vi "Dashboard Main.vi"() -> ()   [LabVIEW 2016]
uses:
  <vilib>/Utility/miscctls.llb/LVRowAndColumnTypeDef.ctl
  <vilib>/event_ctls.llb/eventvkey.ctl
  <vilib>/Rock Robotics/Network Tables/NT Read Boolean.vi
  <vilib>/Rock Robotics/WPI/Dashboard/WPI_DashboardLogging Global.vi
panel:
  out "timeLeft":dbl(slide) scale=0.0..150.0
  in  "TCP":refnum<k5>
  in  "Rec Mode":enum32{"Stop", "Record", "Playback"}(radio)
  out "Robot IP":string
  out "Image Message":string="Timeout in Camera Communications"
  in  "Dashboard Tab":T1(tab)
  out "Angle":dbl(knob) scale=-30.0..30.0
  out "Distance":dbl(slide)
  out "Shooter Speed":dbl(knob) scale=0.0..5600.0
  out "Climber State":u32(colorbox)
  out "Pressure":dbl(knob) scale=0.0..120.0
  out "NT Connection":bool
  out "Mode":T2(ring)=enum."Auto Disabled"
  out "Camera Info":cluster{"Mbps LED":bool, "Mbps":dbl, "fps":dbl} {"fps" format="%#.1g"; "Mbps" format="%#.1g"}
  in  "Autonomous Mode":i32(listbox)
  in  "Peg Side":i32(listbox)
  in  "RPM setting":dbl=5400.0
  out "gearLiftUp":bool
  out "gearLiftDown":bool
  out "gearClawOpen":bool
  out "Camera Image Right":T3(plugin-control)
  in  "DB/String 9":string
  in  "DB/String 8":string
  in  "DB/String 7":string
  in  "DB/String 6":string
  in  "DB/String 5":string
  in  "DB/String 4":string
  in  "DB/String 3":string
  in  "DB/String 2":string
  in  "DB/String 1":string
  in  "DB/String 0":string
  in  "DB/Slider 0":dbl(slide) scale=0.0..5.0
  in  "DB/Slider 1":dbl(slide) scale=0.0..5.0
  in  "DB/Slider 2":dbl(slide) scale=0.0..5.0
  in  "DB/Slider 3":dbl(slide) scale=0.0..5.0
  out "DB/LED 3":bool
  out "DB/LED 2":bool
  out "DB/LED 1":bool
  out "DB/LED 0":bool
  in  "DB/Button 3":bool
  in  "DB/Button 2":bool
  in  "DB/Button 1":bool
  in  "DB/Button 0":bool caption="New Name"
  in  "Camera Name":string(combo)="No Camera Selection"
  in  "Camera Settings":T4={"Frame Rate"=30, "Compression"=30, "Size"=1, "DB Camera Config"=FALSE} {"Frame Rate" scale=1.0..30.0; "Compression" scale=100.0..-1.0; "Size" items=["640x480", "320x240", "160x120"]}
  in  "Camera Name Right":string(combo)="No Camera Selection"
  in  "Camera Settings Right":T4={"Frame Rate"=30, "Compression"=30, "Size"=1, "DB Camera Config"=FALSE} {"Frame Rate" scale=1.0..30.0; "Compression" scale=100.0..-1.0; "Size" items=["640x480", "320x240", "160x120"]}
  in  "Test Slider":dbl(slide) scale=0.0..100.0 scale format="%#_3g"
  in  "On/Off":bool caption="Solenoid"
  in  "Test Name":u16(ring) items=["Select the test to run..."]
  in  "Test Tree":string(tree)
  in  "Motor":cluster{"Value":dbl, "Enable":bool} {"Value" scale=-1.0..1.0 scale format="%#_3g"}
  out "Progress":T5 {"Test Progress" scale=0.0..100.0}
  in  "Rev/Fwd":cluster{"Forward":bool, "Reverse":bool}
  in  "Test Ring":u16(ring) items=["Monochrome", "Color"]
  out "Cmd Status":string
  in  "Execute Command":bool
  in  "Command Params":string[][](table)
  in  "Command Selection":i32(listbox)
  in  "CheckList":i32(listbox)
  out "Tree":string(tree)
  out "Camera Image":T3(plugin-control)
  out "Background":bool
  # "Gear Claw"
  # "HW"
  # "HW"
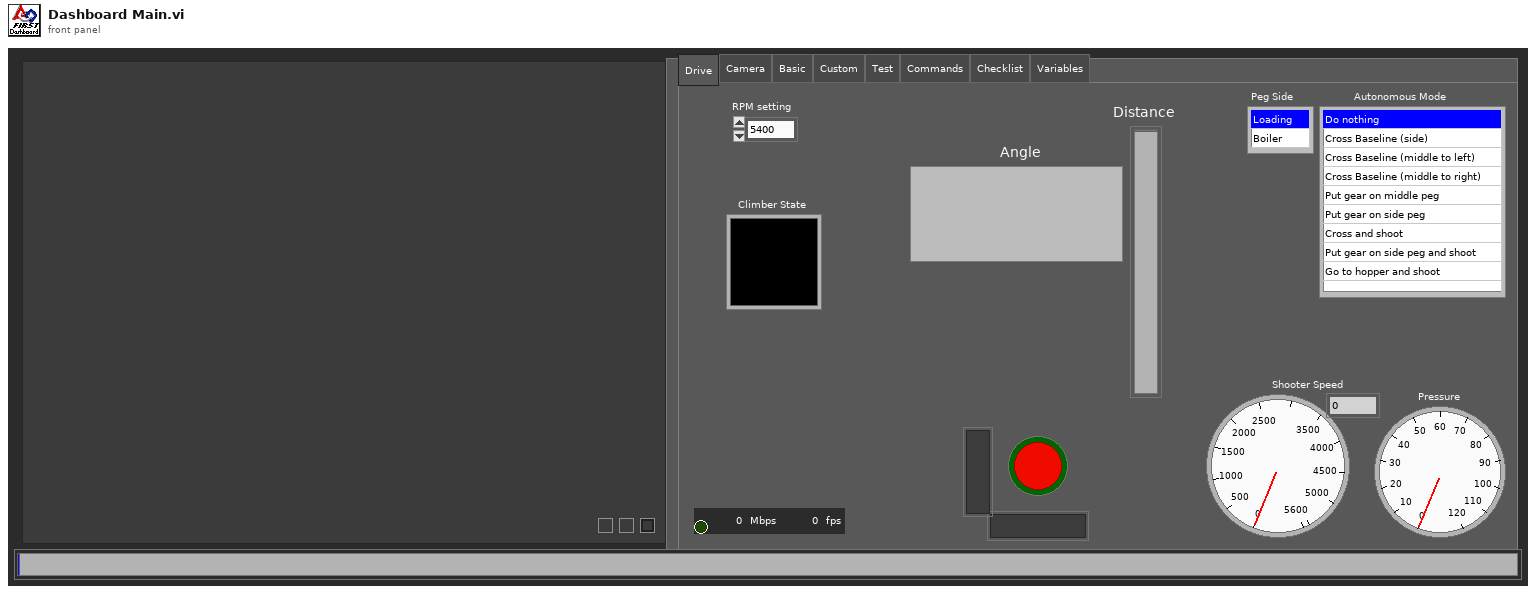
[diagram p1: front panel]
types:
  T1 = enum32{"Drive", "Camera", "Basic", "Custom", "Test", "Commands", "Checklist", "Variables"}
  T2 = enum8{"Tele-Op Disabled", "Tele-Op Enabled", "Auto Disabled", "Auto Enabled", "Test Disabled", "Test Enabled", "Disconnected", "No Code", "E-Stop"}
  T3 = typedef "IMAQ Image.ctl" = refnum<image>
  T4 = cluster{"Frame Rate":i32, "Compression":i32, "Size":u16, "DB Camera Config":bool}
  T5 = cluster{"Test Progress":u8, "Test Progress Text":string}
  T6 = typedef "Image Type" = u32
  T7 = cluster{"IDs":cluster{"RPC field ID":u16, "Unique ID":u16}, "String":string}
  T8 = enum32{"Drive", "Basic", "Custom", "Test", "Checklist", "Variables"}
  T9 = cluster{"Error Strings":string, "Disable Counts":cluster{u16, u16}, "Rail Faults":cluster{u16, u16, u16}, "Robot IP":string, "DB Mode":u8, "Event Info":cluster{"Name":string, "Type":u8, "Number":u16, "Replay":u8}}
  T10 = cluster{"Storage":cluster{"Disk Free":u64, "RAM Block":u32, "RAM free":u32}, "CPU Utilization":cluster{"CPU % ISR":sgl, "CPU % Time Crit":sgl, "CPU % Timed Str":sgl, "CPU % High":sgl, "CPU % Above":sgl, "CPU % Normal":sgl, "CPU % Low":sgl}, "CAN":cluster{"% Bus Utilization":sgl, "Bus Off Cnt":u32, "TX_FIFO Full Cnt":u32, "Receive Error Cnt":u8, "Transmit Error Cnt":u8}, "HID":cluster{"HID Outputs":u32, "Rumble Low":u16, "Rumble High":u16}[]}
  T11 = cluster{"Status bits":cluster{"Test Mode":bool, "Autonomous":bool, "Enabled":bool, "Code Start":bool, "Brownout":bool, "Reserved 2":bool, "Reserved 3":bool, "E-Stop":bool}, "Code Trace":cluster{"Disabled":bool, "TeleOp":bool, "Auto":bool, "Test":bool}, "Controller Type":enum16{"unknown", "cRIO", "roboRio"}, "Code?":enum16{"unknown", "noCode", "code"}, "Battery V":dbl}
  T12 = cluster{"Control Bits":cluster{"TestMode":bool, "Autonomous":bool, "Enabled":bool, "FMS Present":bool, bool, bool, bool, "E-Stop":bool}, "Team Station ":u8, "Countdown":sgl, "Joystick Values":cluster{"Axes":dbl[], "Buttons":bool[], "POVs":i16[]}[]}
  T13 = cluster{"Camera Image":refnum<vi>, "Dashboard Tab":refnum<vi>, "Background":refnum<vi>, "Rec Mode":refnum<vi>, "Test Slider":refnum<vi>, "On/Off ":refnum<vi>, "Test Ring":refnum<vi>, "Rev/Fwd":refnum<vi>, "Test Name":refnum<vi>, "Motor":refnum<vi>, "Progress":refnum<vi>, "CheckList":refnum<vi>, "Tree":refnum<vi>, "Test Tree":refnum<vi>, "Command Params":refnum<vi>, "Command Selection":refnum<vi>, "Execute Command":refnum<vi>, "Cmd Status":refnum<vi>, "Camera Settings":refnum<vi>, "Camera Name":refnum<vi>, "Camera Info":refnum<vi>, "Camera Settings Right":refnum<vi>, "Camera Name Right":refnum<vi>, "Camera Image Right":refnum<vi>}
  T14 = cluster{"Operation":enum16{"Update", "Clear"}, "Color Box":u32}[]
  T15 = typedef "eventvkey.ctl" = enum16{"ASCII", "Enter", "Return", "Shift", "Ctrl", "Alt", "Cmd", "Opt", "Caps", "NumLock", "Clear", "Break", "Up", "Down", "Left", "Right", "Insert", "Delete", "Home", "End", "PageUp", "PageDown", "Escape", "Help", "Pause", "ScrollLock", "F1", "F2", "F3", "F4", "F5", "F6", "F7", "F8", "F9", "F10", "F11", "F12", "F13", "F14", "F15", "F16", "F17", "F18", "F19", "F20", "F21", "F22", "F23", "F24", "Play", "VolumeUp", "VolumeDown", "Mute", "Two Byte Char"}
  T16 = cluster{"Image Size":bool, "Image Type":bool, "Pixel Value":bool, "ROI Information":bool, "Zoom Factor":bool}
  T17 = cluster{"Operation":enum16{"Update", "Clear"}, "Color Box":u32}
  T18 = typedef "LVRowAndColumnTypeDef.ctl" = cluster{"Row":i32, "Column":i32}
  T19 = cluster{"Shift":bool, "Ctrl":bool, "Alt":bool, "Cmd":bool, "Opt":bool}
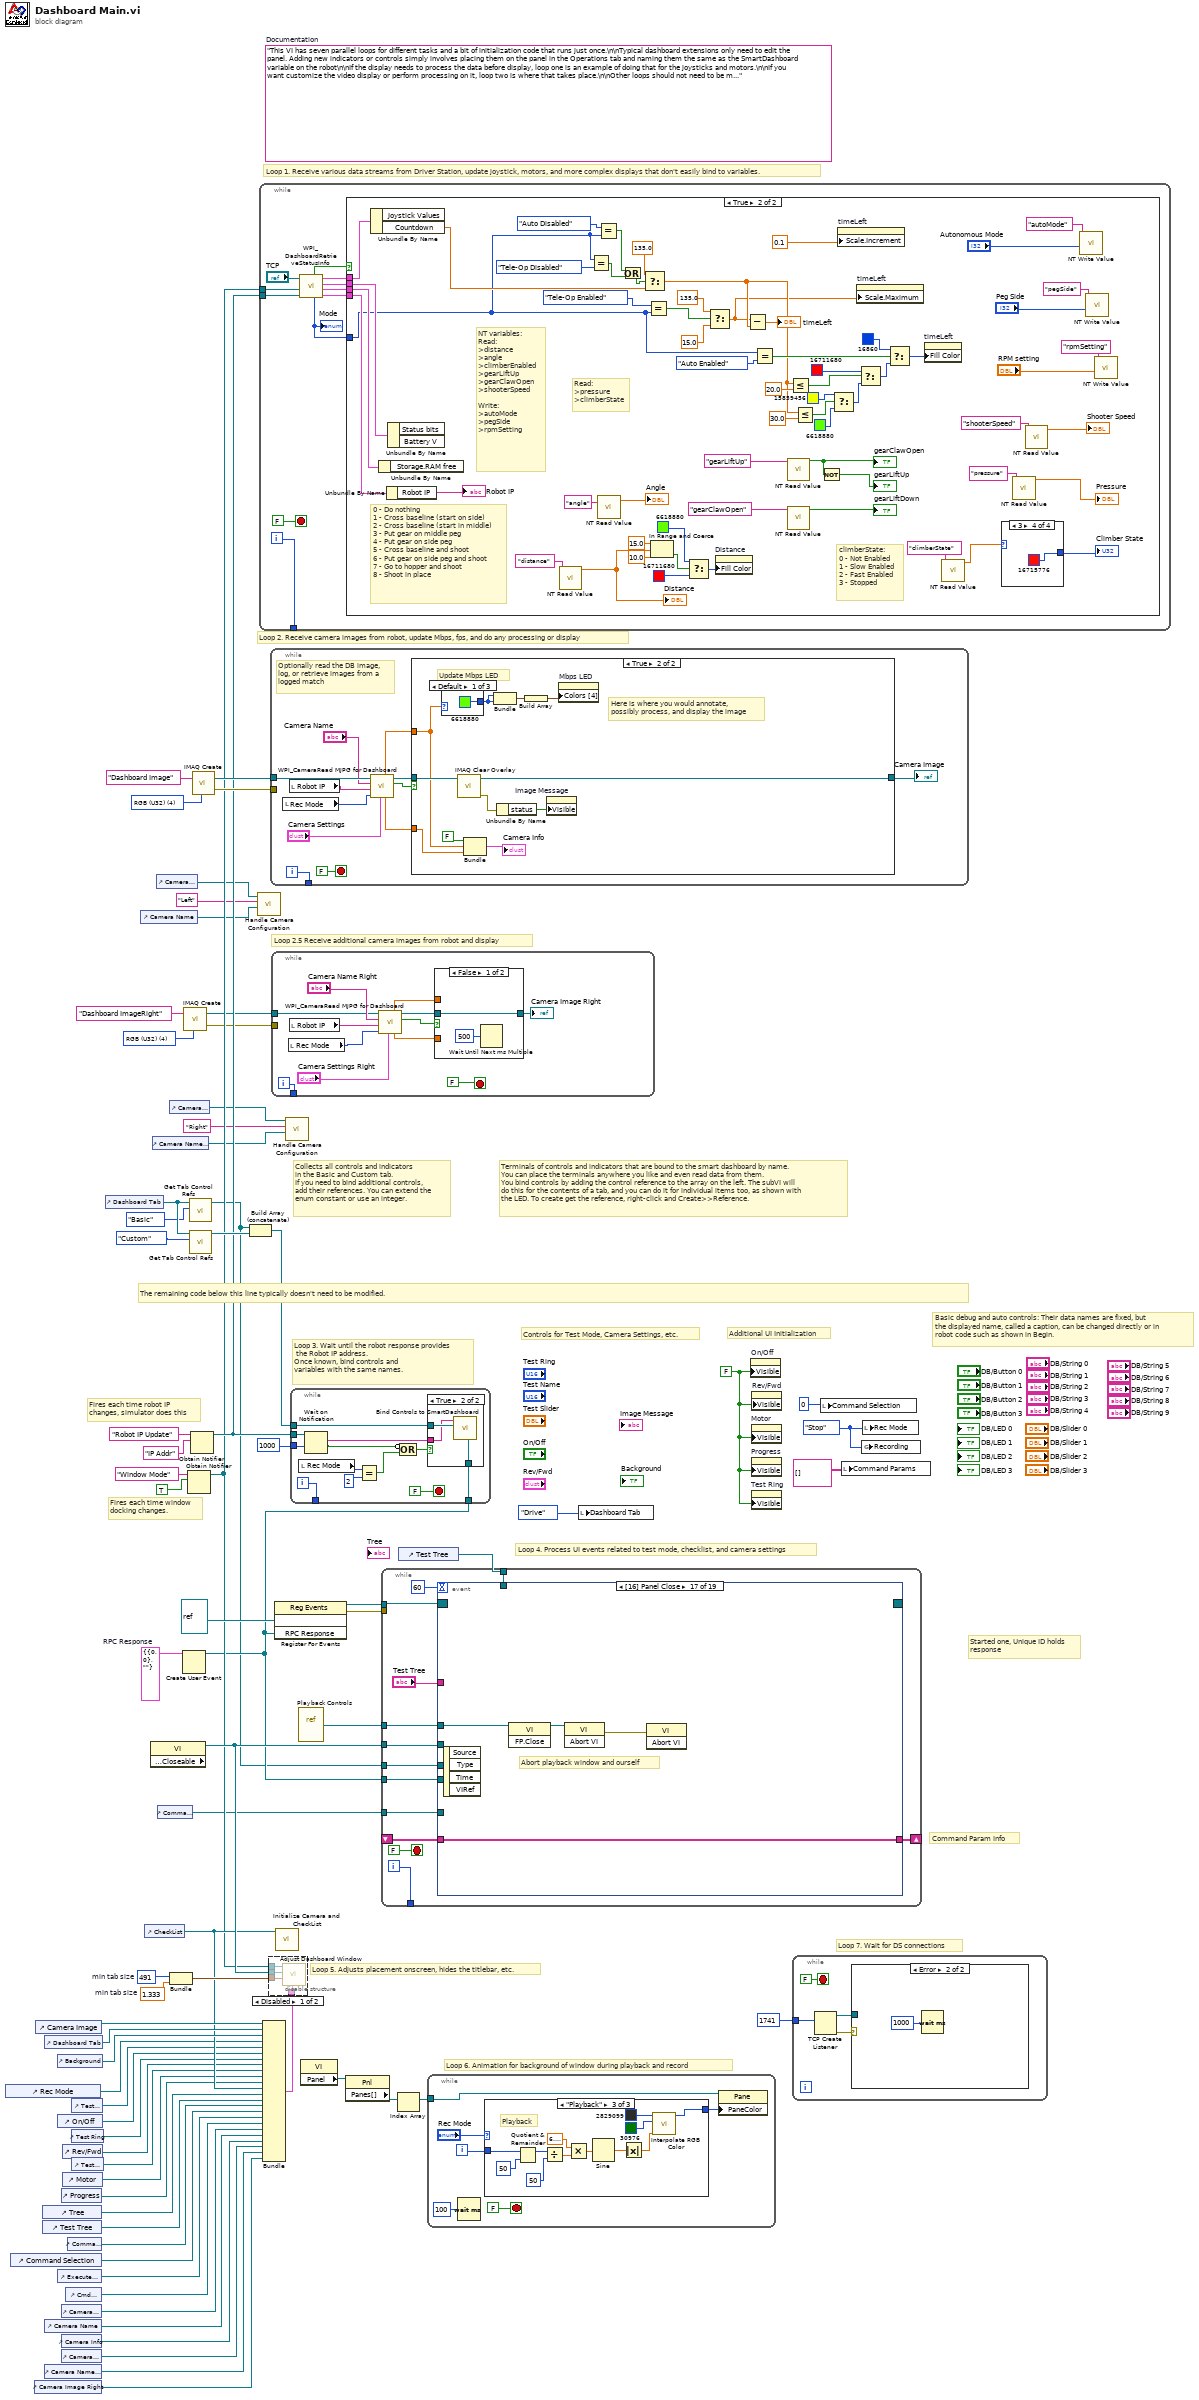
[diagram p0: block diagram]
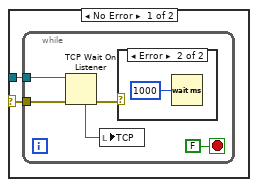
[diagram p4: hidden frame]
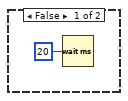
[diagram p6: hidden frame]
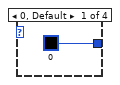
[diagram p7: hidden frame]
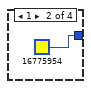
[diagram p8: hidden frame]
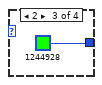
[diagram p9: hidden frame]
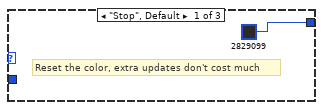
[diagram p10: hidden frame]
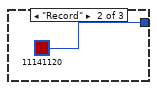
[diagram p11: hidden frame]
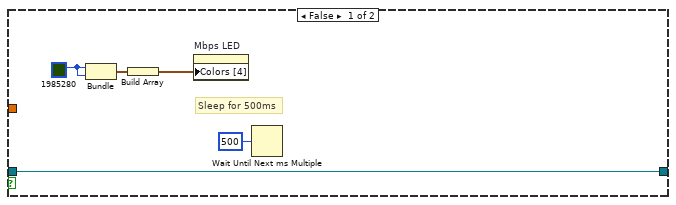
[diagram p13: hidden frame]
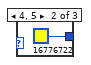
[diagram p14: hidden frame]
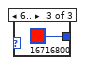
[diagram p15: hidden frame]
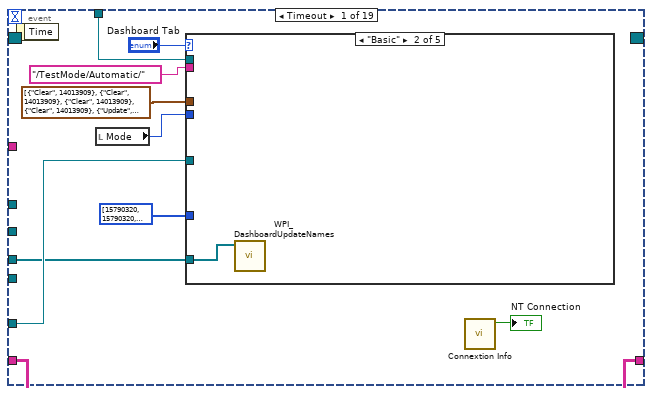
[diagram p16: hidden frame]
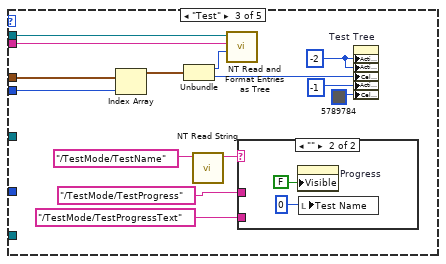
[diagram p18: hidden frame]
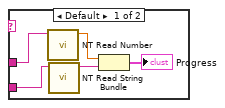
[diagram p19: hidden frame]
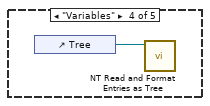
[diagram p20: hidden frame]
diagram:
  w10 = T6 4 items=["Grayscale (U8)", "Grayscale (I16)", "Grayscale (SGL)", "Complex (CSG)", "RGB (U32)", "HSL (U32)", "RGB (U64)"] ("Image Type")
  w24 = T7 {"IDs"={"RPC field ID"=0, "Unique ID"=0}, "String"=""}  # RPC Response
  w49 = 491  # min tab size
  w48 = 1.333  # min tab size
  w56 = enum32{"Stop", "Record", "Playback"}."Stop" ("Rec Mode")
  w31 = FALSE ("Visible")
  (unwired) "This VI has seven parallel loops for different tasks and a bit of initialization code that runs just once.\n\nTypical dashboard extensions only need to edit the panel. Adding new indicators or controls simply involves placing them on the panel in the Operations tab and naming them the same as the SmartDashboard variable on the robot\n\nIf the display needs to process the data before display, loop one is an example of doing that for the joysticks and motors.\n\nIf you want customize the video display or perform processing on it, loop two is where that takes place.\n\nOther loops should not need to be modified. They are pretty standard, and document the task they perform."  # Documentation
  w73 = T6 4 items=["Grayscale (U8)", "Grayscale (I16)", "Grayscale (SGL)", "Complex (CSG)", "RGB (U32)", "HSL (U32)", "RGB (U64)"] ("Image Type")
  # "Loop 2.5 Receive additional camera images from robot and display"
  # "Command Param Info"
  # "Started one, Unique ID holds\nresponse"
  # "Loop 7. Wait for DS connections"
  # "Basic debug and auto controls: Their data names are fixed, but\nthe displayed name, called a caption, can be changed directly or in\nrobot code such as shown in Begin."
  # "Controls for Test Mode, Camera Settings, etc."
  # "Additional UI Initialization"
  # "Loop 6. Animation for background of window during playback and record"
  # "Fires each time robot IP\nchanges, simulator does this"
  # "Fires each time window\ndocking changes."
  # "Collects all controls and indicators\nin the Basic and Custom tab.\nIf you need to bind additional controls,\nadd their references. You can extend the\nenum constant or use an integer."
  # "The remaining code below this line typically doesn't need to be modified."
  # "Loop 4. Process UI events related to test mode, checklist, and camera settings"
  # "Terminals of controls and indicators that are bound to the smart dashboard by name.\nYou can place the terminals anywhere you like and even read data from them.\nYou bind controls by adding the control reference to the array on the left. The subVI will\ndo this for the contents of a tab, and you can do it for individual items too, as shown with\nthe LED. To create get the reference, right-click and Create>>Reference."
  # "Loop 3. Wait until the robot response provides\n the Robot IP address.\nOnce known, bind controls and\nvariables with the same names."
  # "Loop 5. Adjusts placement onscreen, hides the titlebar, etc."
  # "Loop 1. Receive various data streams from Driver Station, update joystick, motors, and more complex displays that don't easily bind to variables."
  # "Loop 2. Receive camera images from robot, update Mbps, fps, and do any processing or display"
  n1 = control-ref of="Rec Mode"() -> (w37:refnum<vi>)
  n2 = control-ref of="Command Selection"() -> (w23:refnum<vi>)
  n3 = control-ref of="Camera Image Right"() -> (w1:refnum<vi>)
  n4 = control-ref of="Camera Image"() -> (w51:refnum<vi>)
  n5 = control-ref of="Tree"() -> (w41:refnum<vi>)
  n6 = control-ref of="Test Tree"() -> (w40:refnum<vi>)
  n7 = control-ref of="Dashboard Tab"() -> (w50:refnum<vi>)
  n8 = control-ref of="Camera Name"() -> (w14:refnum<vi>)
  n9 = control-ref of="Camera Name Right"() -> (w2:refnum<vi>)
  n10 = control-ref of="Execute Command"() -> (w25:refnum<vi>)
  n11 = control-ref of="Background"() -> (w46:refnum<vi>)
  n12 = control-ref of="On/Off"() -> (w35:refnum<vi>)
  n13 = control-ref of="Progress"() -> (w32:refnum<vi>)
  n14 = control-ref of="Camera Settings"() -> (w15:refnum<vi>)
  n15 = control-ref of="Camera Info"() -> (w13:refnum<vi>)
  n16 = control-ref of="Camera Settings Right"() -> (w3:refnum<vi>)
  n17 = control-ref of="Rev/Fwd"() -> (w33:refnum<vi>)
  n18 = control-ref of="Motor"() -> (w38:refnum<vi>)
  n19 = control-ref of="Cmd Status"() -> (w19:refnum<vi>)
  n20 = control-ref of="Command Params"() -> (w26:refnum<vi>)
  n21 = control-ref of="Test Slider"() -> (w36:refnum<vi>)
  n22 = control-ref of="Test Ring"() -> (w34:refnum<vi>)
  n23 = control-ref of="Test Name"() -> (w39:refnum<vi>)
  n24 = control-ref of="Dashboard Tab"() -> (w54:refnum<vi>)
  n25 = control-ref of="Camera Name"() -> (w16:refnum<vi>)
  n26 = control-ref of="CheckList"() -> (w42:refnum<vi>)
  n27 = property class="VI" props=["Front Panel.Closeable"]() -> (reference out=w55:refnum<vi>)  [unwired: 2 in, 2 out]
  n28 = control-ref of="Camera Name Right"() -> (w6:refnum<vi>)
  n29 = control-ref of="Camera Settings"() -> (w17:refnum<vi>)
  n30 = control-ref of="Command Params"() -> (w18:refnum<vi>)
  n31 = control-ref of="Camera Settings Right"() -> (w7:refnum<vi>)
  n32 = Bundle("min tab size"=w49, "min tab size"=w48) -> (w47:cluster{"min tab size":i32, "min tab size":dbl})  [unwired: 1 in]
  n33 = Create User Event(user event datatype=w24) -> (user event=w20:refnum<user-event>)  [unwired: 1 in, 1 out]
  n34 = call "IMAQ Create"("Image Name"="Dashboard ImageRight", "Image Type"=w10) -> ("New Image"=w9:T3, "error out"=w8:errorcluster)  [unwired: 2 in, 1 out]
  n35 = Obtain Notifier(name (unnamed)="Window Mode", notification data type=TRUE) -> (notifier out=w29:refnum<notifier>)  [unwired: 2 in, 2 out]
  n36 = call <vilib>:"Get Tab Control Refs.vi"("Page Index"=T8."Basic" ("Dashboard Tab"), "TabControl in"=w54) -> ("ControlsOnPage"=w12:refnum<vi>[])  [unwired: 9 in]
  n37 = call <vilib>:"Get Tab Control Refs.vi"("Page Index"=T8."Custom" ("Dashboard Tab"), "TabControl in"=w54) -> ("ControlsOnPage"=w53:refnum<vi>[])  [unwired: 9 in]
  n38 = Obtain Notifier(name (unnamed)="Robot IP Update", notification data type="IP Addr" ("name (unnamed)")) -> (notifier out=w30:refnum<notifier>)  [unwired: 2 in, 2 out]
  n39 = call "IMAQ Create"("Image Name"="Dashboard Image", "Image Type"=w73) -> ("New Image"=w71:T3, "error out"=w70:errorcluster)  [unwired: 2 in, 1 out]
  n40 = Build Array (concatenate)(w12, w53) -> (w52:refnum<vi>[])
  n41 = call "Handle Camera Configuration.vi"("CameraNameRef"=w16, "Camera File Name"="Left", "ClusterRef"=w17) -> ()  [unwired: 9 in]
  n42 = while {
    tunnel: [w83] -> _
    tunnel: w30 -> [w77]
    tunnel: w29 -> [w74]
    i -> [w83]
    stop <- FALSE stop-if-true
    n43 = call <vilib>:"WPI_DashboardRetrieveStatusInfo.vi"("Binding Refnum"=w77, "Window Mode Notifier"=w74, "TCP Cnx"="TCP") -> ("Power and Errors"=w78:T9, "Robot Metrics"=w81:T10, "Status Info"=w82:T11, "Control Info"=w79:T12, "Robot Mode"=w76:T2, "Process?"=w80:bool)  [unwired: 3 in]
    "Mode" <- w76
    n44 = case shown="True" w80 {
      tunnel: w82 -> [_ w147]
      tunnel: w81 -> [_ w146]
      tunnel: w79 -> [_ w145]
      tunnel: w78 -> [_ w144]
      tunnel: w76 -> [_ w114]
      frame False {
        n45 = Wait (ms)(milliseconds to wait=u32 20) -> ()  [unwired: 1 out]
      }
      frame True {
        # "climberState:\n0 - Not Enabled\n1 - Slow Enabled\n2 - Fast Enabled\n3 - Stopped"
        # "Read:\n>pressure\n>climberState"
        # "0 - Do nothing\n1 - Cross baseline (start on side)\n2 - Cross baseline (start in middle)\n3 - Put gear on middle peg\n4 - Put gear on side peg\n5 - Cross baseline and shoot\n6 - Put gear on side peg and shoot\n7 - Go to hopper and shoot\n8 - Shoot in place"
        # "NT variables:\nRead:\n>distance\n>angle\n>climberEnabled\n>gearLiftUp\n>gearClawOpen\n>shooterSpeed\n\nWrite:\n>autoMode\n>pegSide\n>rpmSetting"
        n46 = Unbundle By Name(w145) -> ("Countdown"=w115:sgl)  [unwired: 1 out]
        n47 = Unbundle By Name(w146) -> ()  [unwired: 1 out]
        n48 = Unbundle By Name(w144) -> ("Robot IP"=→"Robot IP":string)
        n49 = Unbundle By Name(w147) -> ()  [unwired: 2 out]
        n50 = call-poly <vilib>:"NT Read Value.vi"("Name"="distance") -> ("Numeric"=w90:dbl)  [unwired: 9 in, 1 out]
        "Distance" <- w90
        n51 = Equal?(x=w114, y=T2."Tele-Op Disabled") -> (x = y?=w118:bool)
        n52 = Equal?(x=T2."Auto Disabled" ("Robot Mode"), y=w114) -> (x = y?=w119:bool)
        n53 = call-poly <vilib>:"NT Read Value.vi"("Name"="angle") -> ("Numeric"=→"Angle":dbl)  [unwired: 9 in, 1 out]
        n54 = Or(x=w119, y=w118) -> (x .or. y?=w120:bool)
        n55 = Select(t=sgl 135.0, s=w120, f=w115) -> (s? t:f=w124:sgl)
        n56 = Equal?(x=T2."Tele-Op Enabled" ("Robot Mode"), y=w114) -> (x = y?=w126:bool)
        n57 = In Range and Coerce(upper limit=15.0, x=w90, lower limit=10.0) -> (In Range?=w93:bool)  [unwired: 1 out]
        n58 = Select(t=u32 6618880, s=w93, f=u32 16711680) -> (s? t:f=w94:u32)
        n59 = Select(t=135.0, s=w126, f=15.0) -> (s? t:f=w122:dbl)
        n60 = property on="Distance" class="Slide (strict)"("Fill Color"=w94) -> ()  [unwired: 2 in, 2 out]
        n61 = Subtract(x=w122, y=w124) -> (x-y=→"timeLeft":dbl)
        n62 = Equal?(x=w114, y=T2."Auto Enabled") -> (x = y?=w137:bool)
        n63 = call-poly <vilib>:"NT Read Value.vi"("Name"="gearLiftUp") -> ("Boolean"=w98:bool)  [unwired: 9 in, 1 out]
        "gearClawOpen" <- w98
        n64 = call-poly <vilib>:"NT Read Value.vi"("Name"="gearClawOpen") -> ("Boolean"=→"gearLiftDown":bool)  [unwired: 9 in, 1 out]
        n65 = Less Or Equal?(x=w124, y=sgl 20.0) -> (x <= y?=w116:bool)
        n66 = Less Or Equal?(x=w124, y=sgl 30.0) -> (x <= y?=w129:bool)
        n67 = Not(x=w98) -> (.not. x?=→"gearLiftUp":bool)
        n68 = Select(t=u32 15859456, s=w129, f=u32 6618880) -> (s? t:f=w130:u32)
        n69 = property on="timeLeft" class="Slide (strict)"("Scale.Increment"=0.1 ("Scale.Range:Increment")) -> ()  [unwired: 2 in, 2 out]
        n70 = property on="timeLeft" class="Slide (strict)"("Scale.Maximum"=w122) -> ()  [unwired: 2 in, 2 out]
        n71 = Select(t=u32 16711680, s=w116, f=w130) -> (s? t:f=w132:u32)
        n72 = Select(t=u32 16860, s=w137, f=w132) -> (s? t:f=w135:u32)
        n73 = property on="timeLeft" class="Slide (strict)"("Fill Color"=w135) -> ()  [unwired: 2 in, 2 out]
        n74 = call-poly <vilib>:"NT Read Value.vi"("Name"="climberState") -> ("Numeric"=w106:dbl)  [unwired: 9 in, 1 out]
        n75 = case shown="3" w106 {
          tunnel: [u32 0 ("Climber State") u32 16775954 ("Climber State") u32 1244928 ("Climber State") u32 16715776 ("Climber State")] -> w105
          frame 0, Default {
          }
          frame 1 {
          }
          frame 2 {
          }
          frame 3 {
          }
        }
        "Climber State" <- w105
        n76 = call-poly <vilib>:"NT Read Value.vi"("Name"="pressure") -> ("Numeric"=→"Pressure":dbl)  [unwired: 9 in, 1 out]
        n77 = call-poly <vilib>:"NT Read Value.vi"("Name"="shooterSpeed") -> ("Numeric"=→"Shooter Speed":dbl)  [unwired: 9 in, 1 out]
        n78 = call-poly <vilib>:"NT Write Value.vi"("Numeric"="Autonomous Mode", "Name"="autoMode") -> ()  [unwired: 9 in, 1 out]
        n79 = call-poly <vilib>:"NT Write Value.vi"("Numeric"="Peg Side", "Name"="pegSide") -> ()  [unwired: 9 in, 1 out]
        n80 = call-poly <vilib>:"NT Write Value.vi"("Numeric"="RPM setting", "Name"="rpmSetting") -> ()  [unwired: 9 in, 1 out]
      }
    }
  }
  n81 = Bundle("Camera Image"=w51, "Dashboard Tab"=w50, "Background"=w46, "Rec Mode"=w37, "Test Slider"=w36, "On/Off"=w35, "Test Ring"=w34, "Rev/Fwd"=w33, "Test Name"=w39, "Motor"=w38, "Progress"=w32, "CheckList"=w42, "Tree"=w41, "Test Tree"=w40, "Command Params"=w26, "Command Selection"=w23, "Execute Command"=w25, "Cmd Status"=w19, "Camera Settings"=w15, "Camera Name"=w14, "Camera Info"=w13, "Camera Settings Right"=w3, "Camera Name Right"=w2, "Camera Image Right"=w1) -> (w43:T13)  [unwired: 1 in]
  n82 = disable-structure shown="Disabled" {
    disable-tunnel: w55 -> [w155 _]
    disable-tunnel: w47 -> [w154 _]
    disable-tunnel: w43 -> [w153 _]
    disable-tunnel: w29 -> [w152 _]
    frame Disabled {
      n83 = call "Adjust Dashboard Window.vi"("Sizing Refnums"=w153, "Size Constraints"=w154, "VI"=w155, "WIn Mode"=w152) -> ()  [unwired: 8 in]
    }
    frame Enabled {
    }
  }
  n84 = while {
    tunnel: w71 -> [w165]
    tunnel: w70 -> [_]
    tunnel: [w166] -> _
    i -> [w166]
    stop <- FALSE stop-if-true
    # "Optionally read the DB image,\nlog, or retrieve images from a\nlogged match"
    n85 = local read "Rec Mode"() -> (w161:enum32{"Stop", "Record", "Playback"})
    n86 = local read "Robot IP"() -> (w160:string)
    n87 = call <vilib>:"WPI_CameraRead MJPG for Dashboard.vi"("Camera Settings"="Camera Settings", "Rec Mode"=w161, "Robot IP"=w160, "Camera Name"="Camera Name", "Refnum in"=w165) -> ("Active"=w163:bool, "Refnum out"=w164:T3, "FPS"=w162:dbl, "Bandwidth (Mbps)"=w159:dbl)  [unwired: 3 in]
    n88 = case shown="True" w163 {
      tunnel: w164 -> [w168 w179]
      tunnel: w159 -> [_ w176]
      tunnel: w162 -> [_ w177]
      tunnel: [w168 w173] -> w156
      frame False {
        w170 = u32 1985280 ("Color Box")
        # "Sleep for 500ms"
        n89 = Bundle("Color Box"=w170, "Color Box"=w170) -> (w171:cluster{"Color Box":u32, "Color Box":u32})  [unwired: 1 out]
        n90 = Build Array(w171) -> (w169:cluster{"Color Box":u32, "Color Box":u32}[])
        n91 = property on="Mbps LED" class="Bool (strict)"("Colors [4]"=w169) -> ()  [unwired: 2 in, 2 out]
        n92 = Wait Until Next ms Multiple(millisecond multiple=u32 500) -> ()  [unwired: 1 out]
      }
      frame True {
        # "Here is where you would annotate,\npossibly process, and display the image"
        # "Update Mbps LED"
        n93 = case shown="Default" w176 {
          tunnel: [u32 6618880 ("Color Box") u32 16776722 ("Color Box") u32 16716800 ("Color Box")] -> w180
          frame Default {
          }
          frame 4, 5 {
          }
          frame 6.. {
          }
        }
        n94 = call "IMAQ Clear Overlay"("Image"=w179) -> ("error out"=w182:errorcluster, "Image Out"=w173:T3)  [unwired: 2 in, 7 out]
        n95 = Bundle(FALSE, "Bandwidth (Mbps)"=w176, "FPS"=w177) -> (→"Camera Info":cluster{bool, "Bandwidth (Mbps)":dbl, "FPS":dbl})  [unwired: 1 in]
        n96 = Bundle("Color Box"=w180, "Color Box"=w180) -> (w181:cluster{"Color Box":u32, "Color Box":u32})  [unwired: 1 out]
        n97 = Unbundle By Name(w182) -> ("status"=w183:bool)
        n98 = Build Array(w181) -> (w178:cluster{"Color Box":u32, "Color Box":u32}[])
        n99 = property on="Image Message" class="Str"("Visible"=w183) -> ()  [unwired: 2 in, 2 out]
        n100 = property on="Mbps LED" class="Bool (strict)"("Colors [4]"=w178) -> ()  [unwired: 2 in, 2 out]
      }
    }
    "Camera Image" <- w156
  }
  n101 = while {
    tunnel: w9 -> [w197]
    tunnel: w8 -> [_]
    tunnel: [w191] -> _
    i -> [w191]
    stop <- FALSE stop-if-true
    n102 = local read "Rec Mode"() -> (w195:enum32{"Stop", "Record", "Playback"})
    n103 = local read "Robot IP"() -> (w196:string)
    n104 = call <vilib>:"WPI_CameraRead MJPG for Dashboard.vi"("Camera Settings"="Camera Settings Right", "Rec Mode"=w195, "Robot IP"=w196, "Camera Name"="Camera Name Right", "Refnum in"=w197) -> ("Active"=w190:bool, "Refnum out"=w193:T3, "FPS"=w188:dbl, "Bandwidth (Mbps)"=w189:dbl)  [unwired: 3 in]
    n105 = case shown="False" w190 {
      tunnel: w193 -> [w199 w201]
      tunnel: w189 -> [_ _]
      tunnel: w188 -> [_ _]
      tunnel: [w199 w201] -> w187
      frame False {
        n106 = Wait Until Next ms Multiple(millisecond multiple=u32 500) -> ()  [unwired: 1 out]
      }
      frame True {
      }
    }
    "Camera Image Right" <- w187
  }
  n107 = register-events(refnum<vi> refnum, w20) -> (reference out=w60:refnum<event-registration>, error out=w59:errorcluster)  [unwired: 2 in]
  n108 = call "Initialize Camera and CheckList.vi"("ListBox in"=w42) -> ()  [unwired: 11 in]
  n109 = call "Handle Camera Configuration.vi"("CameraNameRef"=w6, "Camera File Name"="Right", "ClusterRef"=w7) -> ()  [unwired: 9 in]
  n110 = while {
    tunnel: w52 -> [w213]
    tunnel: w30 -> [w211]
    tunnel: [w209] -> _
    tunnel: u32 1000 ("milliseconds to wait") -> [w208]
    tunnel: w20 -> [w202]
    i -> [w209]
    stop <- FALSE stop-if-true
    n111 = local read "Rec Mode"() -> (w204:enum32{"Stop", "Record", "Playback"})
    n112 = Wait on Notification(notifier=w211, timeout in ms (-1)=w208) -> (notification=w210:string, timed out?=w206:bool)  [unwired: 2 in, 2 out]
    n113 = Equal?(x=w204, y=u16 2 ("Rec Mode")) -> (x = y?=w205:bool)
    n114 = Compound Arithmetic op=OR(invert w206, w205) -> (w207:bool)
    n115 = case shown="True" w207 {
      tunnel: w213 -> [_ w216]
      tunnel: w210 -> [_ w215]
      tunnel: w202 -> [_ w214]
      frame False {
      }
      frame True {
        n116 = call <vilib>:"Bind Controls to SmartDashboard.vi"("RPC ref"=w214, "Bound Control Refs"=w216, "Server IP Address"=w215) -> ()  [unwired: 9 in]
      }
    }
  }
  n117 = vi-ref "Playback Controls.vi"() -> (w61:refnum<vi>)
  n118 = property class="VI"() -> ("Panel"=w63:refnum<vi>)  [unwired: 2 in, 2 out]
  n119 = property class="Pnl"(reference=w63) -> ("Panes[]"=w64:refnum<vi>[])  [unwired: 1 in, 2 out]
  n120 = Index Array(array=w64) -> (element=w62:refnum<vi>)  [unwired: 1 in]
  n121 = control-ref of="Test Tree"() -> (w65:refnum<vi>)
  n122 = while {
    tunnel: [w226] -> _
    tunnel: w65 -> [w225]
    tunnel: w61 -> [w224]
    tunnel: w60 -> [w223]
    tunnel: w59 -> [_]
    tunnel: w55 -> [w222]
    tunnel: w20 -> [w221]
    tunnel: w18 -> [w220]
    shift-right: [w219] -> _
    shift-left: _ -> [w218]
    tunnel: w12 -> [w217]
    i -> [w226]
    stop <- FALSE stop-if-true
    n123 = event shown="[16] Panel Close" {
      selector: w223 -> [_ _ _ _ _ _ _ _ _ _ _ _ _ _ _ _ _ _ _]
      dyn-events: [_ _ _ _ _ _ _ _ _ _ _ _ _ _ w476 _ _ _ _] -> _
      timeout: u32 60 ("milliseconds to wait") -> [_ _ _ _ _ _ _ _ _ _ _ _ _ _ _ _ _ _ _]
      tunnel: w225 -> [w238 _ _ _ _ _ _ _ _ _ _ _ _ _ _ _ _ _ _]
      tunnel: "Test Tree" -> [_ _ _ _ _ _ _ _ _ w443 w451 w453 w457 w465 _ _ _ _ _]
      tunnel: w224 -> [_ _ _ _ _ _ _ _ _ _ _ _ _ _ w478 _ w496 _ _]
      tunnel: w222 -> [_ _ _ _ _ _ _ _ _ _ _ _ _ _ w474 _ _ _ _]
      tunnel: w221 -> [_ _ _ _ _ _ _ _ _ _ _ _ _ _ w470 _ _ _ _]
      tunnel: w220 -> [w233 _ _ _ w394 _ _ _ _ _ _ _ _ _ _ _ _ _ _]
      tunnel: [w232 w277 w379 w384 w392 w401 w411 w418 w430 w442 w449 w452 w456 w464 w469 w491 w493 w497 w508] -> w219
      tunnel: w218 -> [w232 w277 w379 w384 w392 _ _ w418 w430 w442 w449 w452 w456 w464 w469 w491 w493 w497 w508]
      tunnel: w217 -> [w230 _ _ _ _ _ _ _ _ _ _ _ _ _ _ _ _ _ _]
      event Timeout {
        n124 = event-data() -> ()  [unwired: 1 in, 1 out]
        n125 = local read "Mode"() -> (w235:T2)
        n126 = case shown="\"Basic\"" "Dashboard Tab" {
          tunnel: w238 -> [_ _ w254 _ _]
          tunnel: "/TestMode/Automatic/" ("Name Pattern") -> [_ _ w253 _ _]
          tunnel: T14 [{"Operation"=enum."Clear", "Color Box"=14013909}, {"Operation"=enum."Clear", "Color Box"=14013909}, {"Operation"=enum."Clear", "Color Box"=14013909}, {"Operation"=enum."Clear", "Color Box"=14013909}, {"Operation"=enum."Update", "Color Box"=14013909}, {"Operation"=enum."Update", "Color Box"=16777215}, {"Operation"=enum."Clear", "Color Box"=14013909}, {"Operation"=enum."Clear", "Color Box"=14013909}, {"Operation"=enum."Clear", "Color Box"=14013909}] -> [_ _ w246 _ w270]
          tunnel: w235 -> [_ _ w245 _ w269]
          tunnel: u32[] [15790320, 15790320, 15790320, 15790320, 16777215, 16777215, 15790320, 15790320, 15790320] -> [_ _ _ _ w275]
          tunnel: w233 -> [_ _ _ _ w263]
          tunnel: w230 -> [_ w240 _ _ _]
          frame "Custom", Default {
          }
          frame "Basic" {
            n127 = call <vilib>:"WPI_DashboardUpdateNames.vi"("Controls on Tab"=w240) -> ()  [unwired: 11 in]
          }
          frame "Test" {
            w252 = -2 ("Active Item:Row Number")
            n128 = Index Array(array=w246, index=w245) -> (element=w247:T17)
            n129 = Unbundle(w247) -> ("Operation"=w248:enum16{"Update", "Clear"}, "Color Box"=w249:u32)
            n130 = call <vilib>:"NT Read String.vi"("Name"="/TestMode/TestName") -> ("String"=w243:string)  [unwired: 9 in, 1 out]
            n131 = call <vilib>:"NT Read and Format Entries as Tree.vi"("Operation"=w248, "Name Pattern"=w253, "Tree Refnum"=w254) -> ()  [unwired: 7 in, 2 out]
            n132 = case shown="\"\"" w243 {
              tunnel: "/TestMode/TestProgress" ("Name") -> [w256 _]
              tunnel: "/TestMode/TestProgressText" ("Name") -> [w255 _]
              frame Default {
                n133 = call <vilib>:"NT Read Number.vi"("Name"=w256) -> ("Numeric"=w257:dbl)  [unwired: 9 in, 1 out]
                n134 = call <vilib>:"NT Read String.vi"("Name"=w255) -> ("String"=w258:string)  [unwired: 9 in, 1 out]
                n135 = Bundle("Numeric"=w257, "String"=w258) -> (→"Progress":cluster{"Numeric":dbl, "String":string})  [unwired: 1 in]
              }
              frame "" {
                n136 = property on="Progress" class="Clust (strict)"("Visible"=FALSE) -> ()  [unwired: 2 in, 2 out]
                n137 = local write "Test Name"(u16 0) -> ()
              }
            }
            n138 = property on="Test Tree" class="Tree (strict)"("Active Item Row Number"=w252, "ActiveColNum"=w252, "CellBG"=w249, "Active Item Row Number"=-1 ("Active Item:Row Number"), "CellBG"=u32 5789784 ("Color Box")) -> ()  [unwired: 2 in, 2 out]
          }
          frame "Variables" {
            n139 = control-ref of="Tree"() -> (w262:refnum<vi>)
            n140 = call <vilib>:"NT Read and Format Entries as Tree.vi"("Tree Refnum"=w262) -> ()  [unwired: 9 in, 2 out]
          }
          frame "Commands" {
            w271 = u32 5789784 ("Color Box")
            w272 = T18 {"Row"=-1, "Column"=-2} ("Active Cell:Active Cell")
            w274 = T18 {"Row"=-2, "Column"=-2} ("Active Cell:Active Cell")
            n141 = Index Array(array=w275, index=w269) -> (element=w273:u32)
            n142 = Index Array(array=w270, index=w269) -> (element=w268:T17)
            n143 = Unbundle(w268) -> ("Operation"=w267:enum16{"Update", "Clear"})  [unwired: 1 out]
            n144 = local read "Command Selection"() -> (w266:i32)
            n145 = property on="Command Selection" class="MCListbox (strict)"("ActiveCell"=w274, "CellBG"=w273, "ActiveCell"=w272, "CellBG"=w271) -> ()  [unwired: 2 in, 2 out]
            n146 = call <vilib>:"WPI_DashboardUpdate RPC Info.vi"("Operation"=w267) -> ("update"=w265:bool, "commands"=w264:string[][])  [unwired: 9 in]
            n147 = property on="Command Selection" class="MCListbox (strict)"("ItemNames"=w264) -> ()  [unwired: 2 in, 2 out]
            n148 = property on="Command Params" class="Tbl (strict)"("Active Cell"=w274, "Cell BG Color"=w273, "Active Cell"=w272, "Cell BG Color"=w271) -> ()  [unwired: 2 in, 2 out]
            n149 = call <vilib>:"WPI_DashboardUpdate Command Params.vi"("Update"=w265, "NewVal"=w266, "Commands"=w264, "Param Tbl"=w263) -> ()  [unwired: 7 in, 1 out]
          }
        }
        n150 = call <vilib>:"Connextion Info.vi"() -> ("Connected"=→"NT Connection":bool)  [unwired: 10 in, 1 out]
      }
      event "Test Tree": Value Change {
        # "Show appropriate\ncontrols"
        n151 = event-data() -> ("CtlRef"=w280:refnum<vi>, "NewVal"=w278:string)  [unwired: 1 in]
        n152 = call <vilib>:"WPI_UtilitiesGetTreeIOName.vi"("NewVal"=w278, "TreeControl in"=w280) -> ("I/O Name"=w281:string)  [unwired: 9 in]
        n153 = case shown="\"Camera\"" w281 {
          selector: w281 -> [_ w288 _ w310 w319 _]
          tunnel: w278 -> [_ _ w307 w309 _ w326]
          tunnel: cluster{string[]}[] [{["640x480", "320x240", "160x120"]}, {["Auto", "Fixed indoor", "Fixed outdoor 1", "Fixed outdoor 2", "Fixed fluorescent 1", "Fixed fluorescent 2", "Hold current"]}, {["Auto", "Flicker-free 50 Hz", "Flicker-free 60 Hz", "Hold current"]}, {["None", "Prioritize frame rate", "Prioritize image quality"]}, {["Monochrome", "Color"]}] -> [_ _ _ _ _ w325]
          frame Default {
            w283 = FALSE ("Visible")
            w282 = FALSE ("Visible")
            n154 = property on="Motor" class="Clust (strict)"("Visible"=w282) -> ()  [unwired: 2 in, 2 out]
            n155 = property on="Test Ring" class="Ring (strict)"("Visible"=w282) -> ()  [unwired: 2 in, 2 out]
            n156 = property on="Rev/Fwd" class="Clust (strict)"("Visible"=w283) -> ()  [unwired: 2 in, 2 out]
            n157 = property on="On/Off" class="Bool (strict)"("Visible"=w283) -> ()  [unwired: 2 in, 2 out]
            n158 = property on="Test Slider" class="Slide (strict)"("Visible"=w283) -> ()  [unwired: 2 in, 2 out]
          }
          frame "Analog Out", "Motor", "PWM" {
            w289 = FALSE ("Visible")
            n159 = case shown="\"Analog Out\"" w288 {
              tunnel: [1.0 ("Value") -1.0 ("Value") 0.0 ("Value")] -> w287
              tunnel: [255.0 ("Value") 1.0 ("Value") 5.0 ("Value")] -> w286
              tunnel: [128.0 ("Value") 0.0 ("Value") 0.0 ("Value")] -> w285
              tunnel: [64.0 ("Value") 0.5 ("Value") 1.0 ("Value")] -> w284
              frame "PWM" {
              }
              frame "Motor", Default {
              }
              frame "Analog Out" {
              }
            }
            n160 = property on="Motor" class="Clust (strict)"("Visible"=TRUE) -> ()  [unwired: 2 in, 2 out]
            n161 = property on="Value" class="Slide (strict)"("Value"=w285, "Scale.Minimum"=w287, "Scale.Maximum"=w286, "Scale.Increment"=w284) -> ()  [unwired: 2 in, 2 out]
            n162 = property on="On/Off" class="Bool (strict)"("Visible"=w289) -> ()  [unwired: 2 in, 2 out]
            n163 = property on="Test Slider" class="Slide (strict)"("Visible"=w289) -> ()  [unwired: 2 in, 2 out]
            n164 = property on="Test Ring" class="Ring (strict)"("Visible"=w289) -> ()  [unwired: 2 in, 2 out]
            n165 = property on="Rev/Fwd" class="Clust (strict)"("Visible"=w289) -> ()  [unwired: 2 in, 2 out]
          }
          frame "Servo" {
            w305 = FALSE ("Visible")
            n166 = call <vilib>:"NT Read Number.vi"("Name"=w307) -> ("Numeric"=w306:dbl)  [unwired: 9 in, 1 out]
            n167 = property on="Test Slider" class="Slide (strict)"("Visible"=TRUE, "Scale.Maximum"=170.0 ("Scale.Range:Maximum")) -> ()  [unwired: 2 in, 2 out]
            n168 = local write "Test Slider"(w306) -> ()
            n169 = property on="Motor" class="Clust (strict)"("Visible"=w305) -> ()  [unwired: 2 in, 2 out]
            n170 = property on="Rev/Fwd" class="Clust (strict)"("Visible"=w305) -> ()  [unwired: 2 in, 2 out]
            n171 = property on="On/Off" class="Bool (strict)"("Visible"=w305) -> ()  [unwired: 2 in, 2 out]
            n172 = property on="Test Ring" class="Ring (strict)"("Visible"=w305) -> ()  [unwired: 2 in, 2 out]
          }
          frame "Relay", "Solenoid" {
            w308 = FALSE ("Visible")
            n173 = property on="Motor" class="Clust (strict)"("Visible"=w308) -> ()  [unwired: 2 in, 2 out]
            n174 = property on="Test Slider" class="Slide (strict)"("Visible"=w308) -> ()  [unwired: 2 in, 2 out]
            n175 = Search and Replace String(input string=w309, search string="/Value  **", replace string="/Direction") -> (result string=w315:string)  [unwired: 5 in, 3 out]
            n176 = property on="Test Ring" class="Ring (strict)"("Visible"=w308) -> ()  [unwired: 2 in, 2 out]
            n177 = call <vilib>:"NT Read String.vi"("Name"=w315) -> ("String"=w313:string)  [unwired: 9 in, 1 out]
            n178 = Equal?(x="Both directions", y=w313) -> (x = y?=w311:bool)
            n179 = Not(x=w311) -> (.not. x?=w312:bool)
            n180 = property on="Rev/Fwd" class="Clust (strict)"("Visible"=w311) -> ()  [unwired: 2 in, 2 out]
            n181 = property on="On/Off" class="Bool (strict)"("Visible"=w312, "Caption.Text"=w310) -> ()  [unwired: 2 in, 2 out]
          }
          frame "Compressor", "Digital Out" {
            w318 = FALSE ("Visible")
            # "Get direction and finish"
            n182 = property on="Motor" class="Clust (strict)"("Visible"=w318) -> ()  [unwired: 2 in, 2 out]
            n183 = property on="Test Slider" class="Slide (strict)"("Visible"=w318) -> ()  [unwired: 2 in, 2 out]
            n184 = property on="Test Ring" class="Ring (strict)"("Visible"=w318) -> ()  [unwired: 2 in, 2 out]
            n185 = property on="On/Off" class="Bool (strict)"("Visible"=TRUE, "Caption.Text"=w319) -> ()  [unwired: 2 in, 2 out]
            n186 = property on="Rev/Fwd" class="Clust (strict)"("Visible"=FALSE) -> ()  [unwired: 2 in, 2 out]
          }
          frame "Camera" {
            n187 = call <vilib>:"Get Last Path Segment.vi"("String in"=w326) -> ("String out"=w327:string)  [unwired: 10 in]
            n188 = property on="On/Off" class="Bool (strict)"("Visible"=FALSE) -> ()  [unwired: 2 in, 2 out]
            n189 = property on="Motor" class="Clust (strict)"("Visible"=FALSE) -> ()  [unwired: 2 in, 2 out]
            n190 = property on="Rev/Fwd" class="Clust (strict)"("Visible"=FALSE) -> ()  [unwired: 2 in, 2 out]
            n191 = case shown="\"White Balance  **\"" w327 {
              tunnel: w326 -> [w333 w342 w351 w360 w369 _ w375]
              tunnel: w325 -> [w331 w339 w348 w357 w366 _ _]
              frame "Size  **" {
                n192 = Index Array(array=w331) -> (element=w330:cluster{string[]})  [unwired: 1 in]
                n193 = call <vilib>:"NT Read String.vi"("Name"=w333) -> ("String"=w332:string)  [unwired: 9 in, 1 out]
                n194 = Unbundle(w330) -> (w328:string[])
                n195 = Match First String(2:w328, 3:w332) -> (0:w329:i32)  [unwired: 1 out]
                n196 = property on="Test Ring" class="Ring (strict)"("Value"=w329, "Strings []"=w328) -> ()  [unwired: 2 in, 2 out]
                n197 = property on="Test Ring" class="Ring (strict)"("Visible"=TRUE) -> ()  [unwired: 2 in, 2 out]
                n198 = property on="Test Slider" class="Slide (strict)"("Visible"=FALSE) -> ()  [unwired: 2 in, 2 out]
              }
              frame "White Balance  **" {
                n199 = Index Array(array=w339, index=1) -> (element=w340:cluster{string[]})
                n200 = call <vilib>:"NT Read String.vi"("Name"=w342) -> ("String"=w341:string)  [unwired: 9 in, 1 out]
                n201 = Unbundle(w340) -> (w337:string[])
                n202 = Match First String(2:w337, 3:w341) -> (0:w336:i32)  [unwired: 1 out]
                n203 = property on="Test Ring" class="Ring (strict)"("Value"=w336, "Strings []"=w337) -> ()  [unwired: 2 in, 2 out]
                n204 = property on="Test Ring" class="Ring (strict)"("Visible"=TRUE) -> ()  [unwired: 2 in, 2 out]
                n205 = property on="Test Slider" class="Slide (strict)"("Visible"=FALSE) -> ()  [unwired: 2 in, 2 out]
              }
              frame "Exposure  **" {
                n206 = Index Array(array=w348, index=2) -> (element=w349:cluster{string[]})
                n207 = call <vilib>:"NT Read String.vi"("Name"=w351) -> ("String"=w350:string)  [unwired: 9 in, 1 out]
                n208 = Unbundle(w349) -> (w345:string[])
                n209 = Match First String(2:w345, 3:w350) -> (0:w346:i32)  [unwired: 1 out]
                n210 = property on="Test Ring" class="Ring (strict)"("Value"=w346, "Strings []"=w345) -> ()  [unwired: 2 in, 2 out]
                n211 = property on="Test Ring" class="Ring (strict)"("Visible"=TRUE) -> ()  [unwired: 2 in, 2 out]
                n212 = property on="Test Slider" class="Slide (strict)"("Visible"=FALSE) -> ()  [unwired: 2 in, 2 out]
              }
              frame "Exposure Priority  **" {
                n213 = Index Array(array=w357, index=3) -> (element=w358:cluster{string[]})
                n214 = call <vilib>:"NT Read String.vi"("Name"=w360) -> ("String"=w359:string)  [unwired: 9 in, 1 out]
                n215 = Unbundle(w358) -> (w354:string[])
                n216 = Match First String(2:w354, 3:w359) -> (0:w355:i32)  [unwired: 1 out]
                n217 = property on="Test Ring" class="Ring (strict)"("Value"=w355, "Strings []"=w354) -> ()  [unwired: 2 in, 2 out]
                n218 = property on="Test Ring" class="Ring (strict)"("Visible"=TRUE) -> ()  [unwired: 2 in, 2 out]
                n219 = property on="Test Slider" class="Slide (strict)"("Visible"=FALSE) -> ()  [unwired: 2 in, 2 out]
              }
              frame "Color Enable  **" {
                n220 = Index Array(array=w366, index=4) -> (element=w367:cluster{string[]})
                n221 = call <vilib>:"NT Read String.vi"("Name"=w369) -> ("String"=w368:string)  [unwired: 9 in, 1 out]
                n222 = Unbundle(w367) -> (w363:string[])
                n223 = Match First String(2:w363, 3:w368) -> (0:w364:i32)  [unwired: 1 out]
                n224 = property on="Test Ring" class="Ring (strict)"("Value"=w364, "Strings []"=w363) -> ()  [unwired: 2 in, 2 out]
                n225 = property on="Test Ring" class="Ring (strict)"("Visible"=TRUE) -> ()  [unwired: 2 in, 2 out]
                n226 = property on="Test Slider" class="Slide (strict)"("Visible"=FALSE) -> ()  [unwired: 2 in, 2 out]
              }
              frame Default {
                n227 = property on="Test Ring" class="Ring (strict)"("Visible"=FALSE) -> ()  [unwired: 2 in, 2 out]
                n228 = property on="Test Slider" class="Slide (strict)"("Visible"=FALSE) -> ()  [unwired: 2 in, 2 out]
              }
              frame "Brightness  **", "Color Level  **", "Compression  **", "FPS  **", "Sharpness  **" {
                n229 = call <vilib>:"NT Read Number.vi"("Name"=w375) -> ("Numeric"=w374:dbl)  [unwired: 9 in, 1 out]
                n230 = local write "Test Slider"(w374) -> ()
                n231 = property on="Test Slider" class="Slide (strict)"("Visible"=TRUE, "Scale.Maximum"=100.0 ("Scale.Range:Maximum")) -> ()  [unwired: 2 in, 2 out]
                n232 = property on="Test Ring" class="Ring (strict)"("Visible"=FALSE) -> ()  [unwired: 2 in, 2 out]
              }
            }
          }
        }
        n233 = property on="Progress" class="Clust (strict)"("Visible"=FALSE) -> ()  [unwired: 2 in, 2 out]
      }
      event "Test Name": Mouse Enter {
        # "Populate the ring with the list of tests"
        n234 = event-data() -> ()  [unwired: 1 in, 1 out]
        n235 = call <vilib>:"NT Read String Array.vi"("Name"="/TestMode/TestList") -> ("String Array"=w383:string[])  [unwired: 9 in, 1 out]
        n236 = Build Array (concatenate)("Select the test to run...", w383) -> (w382:string[])
        n237 = property on="Test Name" class="Ring (strict)"("Strings []"=w382) -> ()  [unwired: 2 in, 2 out]
      }
      event "Test Name": Value Change {
        w385 = FALSE ("Visible")
        # "Tell the robot the test name to run"
        n238 = event-data() -> ("NewVal"=w389:u16)  [unwired: 1 in]
        n239 = property on="Test Name" class="Ring (strict)"() -> ("Strings []"=w390:string[])  [unwired: 2 in, 2 out]
        n240 = local write "Progress"(T5 {"Test Progress"=0, "Test Progress Text"=""} ("Progress")) -> ()
        n241 = Index Array(array=w390, index=w389) -> (element=w388:string)
        n242 = call <vilib>:"NT Write String.vi"("String"=w388, "Name"="/TestMode/TestName") -> ()  [unwired: 9 in, 1 out]
        n243 = property on="Progress" class="Clust (strict)"("Visible"=TRUE) -> ()  [unwired: 2 in, 2 out]
        n244 = property on="Motor" class="Clust (strict)"("Visible"=w385) -> ()  [unwired: 2 in, 2 out]
        n245 = property on="Test Slider" class="Slide (strict)"("Visible"=w385) -> ()  [unwired: 2 in, 2 out]
        n246 = property on="On/Off" class="Bool (strict)"("Visible"=w385) -> ()  [unwired: 2 in, 2 out]
        n247 = property on="Rev/Fwd" class="Clust (strict)"("Visible"=w385) -> ()  [unwired: 2 in, 2 out]
        n248 = property on="Test Ring" class="Ring (strict)"("Visible"=w385) -> ()  [unwired: 2 in, 2 out]
      }
      event "Command Selection": Value Change {
        # "Get the params and show in table"
        n249 = event-data() -> ("NewVal"=w395:i32)  [unwired: 1 in]
        n250 = property on="Command Selection" class="MCListbox (strict)"() -> ("ItemNames"=w393:string[][])  [unwired: 2 in, 2 out]
        n251 = call <vilib>:"WPI_DashboardUpdate Command Params.vi"("NewVal"=w395, "Commands"=w393, "Param Tbl"=w394) -> ()  [unwired: 8 in, 1 out]
      }
      event "Execute Command": Value Change {
        # "Started one, Unique ID holds\nresponse"
        n252 = event-data() -> ()  [unwired: 1 in, 1 out]
        n253 = property on="Command Selection" class="MCListbox (strict)"() -> ("ItemNames"=w406:string[][])  [unwired: 2 in, 2 out]
        n254 = Index Array(array=w406, index (row)="Command Selection", index (col)=0) -> (element=w404:string)
        n255 = call <vilib>:"Invoke Commands.vi"("Command Params"="Command Params", "Function Name"=w404) -> ("Params"=w400:u8, "Started"=w399:bool)  [unwired: 7 in, 1 out]
        n256 = Array Subset(array="Command Params", length (row)=w400) -> (w401:string[][])  [unwired: 3 in]
        n257 = Select(t="Executing" ("Cmd Status"), s=w399, f="" ("Cmd Status")) -> (s? t:f=→"Cmd Status":string)
      }
      event "Command Selection": Double Click {
        n258 = event-data() -> ("Row"=w414:i32)  [unwired: 1 in]
        n259 = property on="Command Selection" class="MCListbox (strict)"() -> ("ItemNames"=w417:string[][])  [unwired: 2 in, 2 out]
        n260 = local read "Command Params"() -> (w413:string[][])
        n261 = Index Array(array=w417, index (row)=w414, index (col)=0) -> (element=w415:string)
        n262 = call <vilib>:"Invoke Commands.vi"("Command Params"=w413, "Function Name"=w415) -> ("Params"=w412:u8, "Started"=w407:bool)  [unwired: 7 in, 1 out]
        n263 = Array Subset(array=w413, length (row)=w412) -> (w411:string[][])  [unwired: 3 in]
        n264 = Select(t="Executing" ("Cmd Status"), s=w407, f="" ("Cmd Status")) -> (s? t:f=w408:string)
        n265 = local write "Cmd Status"(w408) -> ()
      }
      event "CheckList": Double Click {
        # "Shift clears all"
        # "Update symbols on the listbox"
        n266 = event-data() -> ("PlatMods.Shift"=w419:bool, "Row"=w421:i32)  [unwired: 1 in]
        n267 = case shown="True" w419 {
          tunnel: w421 -> [w425 _]
          tunnel: 1 -> [w424 _]
          frame False {
            n268 = property on="CheckList" class="LstBox (strict)"() -> ("Item Symbols"=w423:i32[])  [unwired: 2 in, 2 out]
            n269 = Replace Array Subset(array=w423, new element=w424, index=w425) -> (w422:i32[])
            n270 = property on="CheckList" class="LstBox (strict)"("Item Symbols"=w422) -> ()  [unwired: 2 in, 2 out]
          }
          frame True {
            w426 = 0 ("Top Row")
            n271 = property on="CheckList" class="LstBox (strict)"() -> ("Number of Rows"=w428:u32)  [unwired: 2 in, 2 out]
            n272 = Initialize Array(0, w428) -> (w427:i32[])
            n273 = property on="CheckList" class="LstBox (strict)"("Top Row"=w426, "Value"=w426, "Item Symbols"=w427) -> ()  [unwired: 2 in, 2 out]
          }
        }
      }
      event "CheckList": Key Down {
        # "Update symbols on the listbox\nLeft and right keys check and uncheck"
        n274 = event-data() -> ("VKey"=w432:T15)  [unwired: 1 in]
        n275 = case shown="\"Left\", \"Right\"" w432 {
          selector: w432 -> [w437 _]
          tunnel: eventvkey."Left" ("VKey") -> [w435 _]
          frame "Left", "Right" {
            n276 = Equal?(x=w435, y=w437) -> (x = y?=w436:bool)
            n277 = Select(t=0, s=w436, f=1) -> (s? t:f=w438:i32)
            n278 = property on="CheckList" class="LstBox (strict)"() -> ("Item Symbols"=w441:i32[])  [unwired: 2 in, 2 out]
            n279 = Replace Array Subset(array=w441, new element=w438, index="CheckList") -> (w440:i32[])
            n280 = property on="CheckList" class="LstBox (strict)"("Item Symbols"=w440) -> ()  [unwired: 2 in, 2 out]
          }
          frame Default {
          }
        }
      }
      event "Motor.Enable": Value Change {
        # "When the test mode otor enable helper is set, update that\ntree row item's value"
        n281 = event-data() -> ("NewVal"=w447:bool)  [unwired: 1 in]
        n282 = Unbundle("Motor") -> ("Value"=w446:dbl)  [unwired: 1 out]
        n283 = Select(t=w446, s=w447, f=0.0) -> (s? t:f=w444:dbl)
        n284 = call <vilib>:"NT Write Number.vi"("Numeric"=w444, "Name"=w443) -> ()  [unwired: 9 in, 1 out]
      }
      event "Test Slider": Value Change {
        # "When the test mode slider helper is set, update that\ntree row item's value"
        n285 = event-data() -> ("NewVal"=w450:dbl)  [unwired: 1 in]
        n286 = call <vilib>:"NT Write Number.vi"("Numeric"=w450, "Name"=w451) -> ()  [unwired: 9 in, 1 out]
      }
      event "On/Off": Value Change {
        # "When the test mode on/off helper value is set, update that\ntree row item's value"
        n287 = event-data() -> ("NewVal"=w455:bool)  [unwired: 1 in]
        n288 = Boolean To (0,1)(Boolean=w455) -> (0, 1=w454:i16)
        n289 = call <vilib>:"NT Write Number.vi"("Numeric"=w454, "Name"=w453) -> ()  [unwired: 9 in, 1 out]
      }
      event "Rev/Fwd": Value Change {
        # "When the test mode helper value for relays is set, update that\ntree row item's value"
        n290 = event-data() -> ("NewVal.Forward"=w463:bool, "NewVal.Reverse"=w462:bool)  [unwired: 1 in]
        n291 = Boolean To (0,1)(Boolean=w463) -> (0, 1=w459:i16)
        n292 = Boolean To (0,1)(Boolean=w462) -> (0, 1=w461:i16)
        n293 = Negate(x=w461) -> (-x=w460:i16)
        n294 = Add(x=w459, y=w460) -> (x+y=w458:i16)
        n295 = call <vilib>:"NT Write Number.vi"("Numeric"=w458, "Name"=w457) -> ()  [unwired: 9 in, 1 out]
      }
      event "Test Ring": Value Change {
        # "When a test mode helper value is selected from the ring,\nset the tree item's variable to the string value"
        n296 = event-data() -> ("NewVal"=w467:u16)  [unwired: 1 in]
        n297 = property on="Test Ring" class="Ring (strict)"() -> ("Strings []"=w468:string[])  [unwired: 2 in, 2 out]
        n298 = Index Array(array=w468, index=w467) -> (element=w466:string)
        n299 = call <vilib>:"NT Write String.vi"("String"=w466, "Name"=w465) -> ()  [unwired: 9 in, 1 out]
      }
      event "Rec Mode": Value Change {
        # "Update globals for recording mode and path to read log from.\nClear when logging and let NetworkTables set path for vision to\nuse."
        n300 = event-data() -> ("NewVal"=w479:enum32{"Stop", "Record", "Playback"})  [unwired: 1 in]
        n301 = global write "WPI_DashboardLogging Global.vi" "Logging Filename"(path "") -> ()
        n302 = global write "WPI_DashboardLogging Global.vi" "Recording"(w479) -> ()
        n303 = case shown="\"Playback\"" w479 {
          tunnel: w478 -> [_ w481 w490]
          tunnel: [_ _ w489] -> w476
          tunnel: [_ _ w488] -> _
          tunnel: w474 -> [_ _ w486]
          tunnel: cluster{i32, i32} {-250, 170} -> [_ _ w485]
          tunnel: [_ _ T16 {"Image Size"=TRUE, "Image Type"=TRUE, "Pixel Value"=TRUE, "ROI Information"=TRUE, "Zoom Factor"=FALSE} ("Image Information Shown:All Elements")] -> w472
          tunnel: [_ _ TRUE ("Zoom Factor")] -> w471
          tunnel: w470 -> [_ _ w482]
          frame Default {
          }
          frame "Stop", "Record" {
            # "Place Window too"
            n304 = invoke class="VI" method="FP.Close"(reference=w481) -> (reference out=w480:refnum<vi>)  [unwired: 2 in, 2 out]
            n305 = invoke class="VI" method="Abort VI"(reference=w480) -> ()  [unwired: 2 in, 3 out]
          }
          frame "Playback" {
            n306 = call "Open Playback Panel.vi"("Offset"=w485, "DB VI Ref"=w486, "Playback in"=w490) -> ("Playback out"=w487:refnum<vi>)  [unwired: 8 in]
            n307 = register-events(w487, w482) -> (reference out=w489:refnum<event-registration>, error out=w488:errorcluster)  [unwired: 2 in]
          }
        }
        n308 = property on="Camera Image" class="ImageControl"("Image Information Shown"=w472, "Image Information Visible"=w471) -> ()  [unwired: 2 in, 2 out]
        n309 = call <vilib>:"WPI_DashboardNT Log FieldName Cache.vi"("Operation"=enum16{"Lookup/Add", "Index", "Clear"}."Clear") -> ()  [unwired: 8 in, 3 out]
      }
      event Panel Close {
        w492 = enum32{"Stop", "Record", "Playback"}."Stop" ("Rec Mode")
        # "Playback window has been closed, abort"
        n310 = event-data() -> ()  [unwired: 1 in, 4 out]
        n311 = local write "Rec Mode"(w492) -> ()
        n312 = global write "WPI_DashboardLogging Global.vi" "Recording"(w492) -> ()
      }
      event Panel Close {
        # "Abort playback window and ourself"
        n313 = event-data() -> ()  [unwired: 1 in, 4 out]
        n314 = invoke class="VI" method="FP.Close"(reference=w496) -> (reference out=w495:refnum<vi>)  [unwired: 2 in, 2 out]
        n315 = invoke class="VI" method="Abort VI"(reference=w495) -> (error out=w494:errorcluster)  [unwired: 2 in, 2 out]
        n316 = invoke class="VI" method="Abort VI"(error in=w494) -> ()  [unwired: 2 in, 3 out]
      }
      event User Event {
        n317 = event-data() -> ("IDs"=w503:cluster{"RPC field ID":u16, "Unique ID":u16}, "String"=w502:string)  [unwired: 1 in]
        n318 = Bundle("IDs"=w503, "String"=w502) -> (w501:T7)  [unwired: 1 in]
        n319 = call <vilib>:"Retrieve RPC Response.vi"("RPC Response"=w501) -> ("Output"=w499:string[][])  [unwired: 10 in]
        n320 = Build Array (concatenate)(w497, w499) -> (w498:string[][])
        n321 = local write "Command Params"(w498) -> ()
        n322 = local write "Cmd Status"("" ("Cmd Status")) -> ()
      }
      event "Tree": Double Click {
        n323 = event-data() -> ("PlatMods"=w507:T19, "Tag"=w506:string)  [unwired: 1 in]
        n324 = Unbundle(w507) -> ("Shift"=w505:bool)  [unwired: 4 out]
        n325 = Not(x=w505) -> (.not. x?=w504:bool)
        n326 = call <vilib>:"NT Update Persistence.vi"("Persistence"=w504, "Name"=w506) -> ()  [unwired: 9 in, 1 out]
      }
    }
  }
  n327 = while {
    tunnel: w62 -> [w510]
    i -> [w513]
    stop <- FALSE stop-if-true
    n328 = Wait (ms)(milliseconds to wait=u32 100) -> ()  [unwired: 1 out]
    n329 = case shown="\"Playback\"" "Rec Mode" {
      tunnel: w513 -> [_ _ w528]
      tunnel: [u32 2829099 ("Base Color") u32 11141120 ("Target Color") w517] -> w509
      frame "Stop", Default {
        # "Reset the color, extra updates don't cost much"
      }
      frame "Record" {
      }
      frame "Playback" {
        # "Playback"
        n330 = Quotient & Remainder(x=w528, y=u32 50 ("milliseconds to wait")) -> (x-y*floor(x/y)=w524:u32)  [unwired: 1 out]
        n331 = Divide(x=w524, y=u32 50 ("milliseconds to wait")) -> (x/y=w521:dbl)
        n332 = Multiply(x=6.283185307179586, y=w521) -> (x*y=w526:dbl)
        n333 = Sine(x=w526) -> (sin(x)=w525:dbl)
        n334 = Absolute Value(x=w525) -> (abs(x)=w518:dbl)
        n335 = call "Interpolate RGB Color.vi"("Proportion"=w518, "Target Color"=u32 30976, "Base Color"=u32 2829099) -> ("Result Color"=w517:u32)  [unwired: 8 in]
      }
    }
    n336 = property class="Pane"(reference=w510, "PaneColor"=w509) -> ()  [unwired: 1 in, 2 out]
  }
  n337 = local write "Dashboard Tab"(T1."Drive" ("Dashboard Tab")) -> ()
  n338 = property on="On/Off" class="Bool (strict)"("Visible"=w31) -> ()  [unwired: 2 in, 2 out]
  n339 = property on="Motor" class="Clust (strict)"("Visible"=w31) -> ()  [unwired: 2 in, 2 out]
  n340 = property on="Progress" class="Clust (strict)"("Visible"=w31) -> ()  [unwired: 2 in, 2 out]
  n341 = property on="Test Ring" class="Ring (strict)"("Visible"=w31) -> ()  [unwired: 2 in, 2 out]
  n342 = property on="Rev/Fwd" class="Clust (strict)"("Visible"=w31) -> ()  [unwired: 2 in, 2 out]
  n343 = while {
    tunnel: u16 1741 ("timeout ms (25000)") -> [w530]
    stop <- FALSE stop-if-true
    n344 = TCP Create Listener(10:w530) -> (0:w529:errorcluster, 3:w531:refnum<k5>)  [unwired: 4 in, 1 out]
    n345 = case shown="Error" w529 {
      selector: w529 -> [w533 _]
      tunnel: w531 -> [w534 _]
      frame No Error {
        n346 = while {
          tunnel: w534 -> [w537]
          tunnel: w533 -> [w536]
          stop <- FALSE stop-if-true
          n347 = TCP Wait On Listener(8:w536, 11:w537) -> (0:w538:errorcluster, 4:w539:refnum<k5>)  [unwired: 2 in, 3 out]
          n348 = local write "TCP"(w539) -> ()
          n349 = case shown="Error" w538 {
            frame No Error {
            }
            frame Error {
              n350 = Wait (ms)(milliseconds to wait=u32 1000) -> ()  [unwired: 1 out]
            }
          }
        }
      }
      frame Error {
        n351 = Wait (ms)(milliseconds to wait=u32 1000) -> ()  [unwired: 1 out]
      }
    }
  }
  n352 = local write "Command Selection"(u16 0 ("milliseconds to wait")) -> ()
  n353 = local write "Command Params"(string[][] [] ("Command Params")) -> ()
  n354 = global write "WPI_DashboardLogging Global.vi" "Recording"(w56) -> ()
  n355 = local write "Rec Mode"(w56) -> ()
